vi "Check Moved File.vi"(7 "Baseline Directory":path, 8 "error in":errorcluster, 10 "Target":string, 11 "File Info in":T1) -> (0 "error out":errorcluster, 3 "File Info out":T1)   [LabVIEW 2020, in "Peer Review.lvclass"]
uses:
  Peer Review.lvclass
  TypeDefs/File Info.ctl
  TypeDefs/File State.ctl
  TypeDefs/VI Type.ctl
  <vilib>/security/Message Digest/API/Instances/File/SHA-256 File Checksum.vi
  <vilib>/security/Message Digest/API/NI_Message Digest API.lvlib
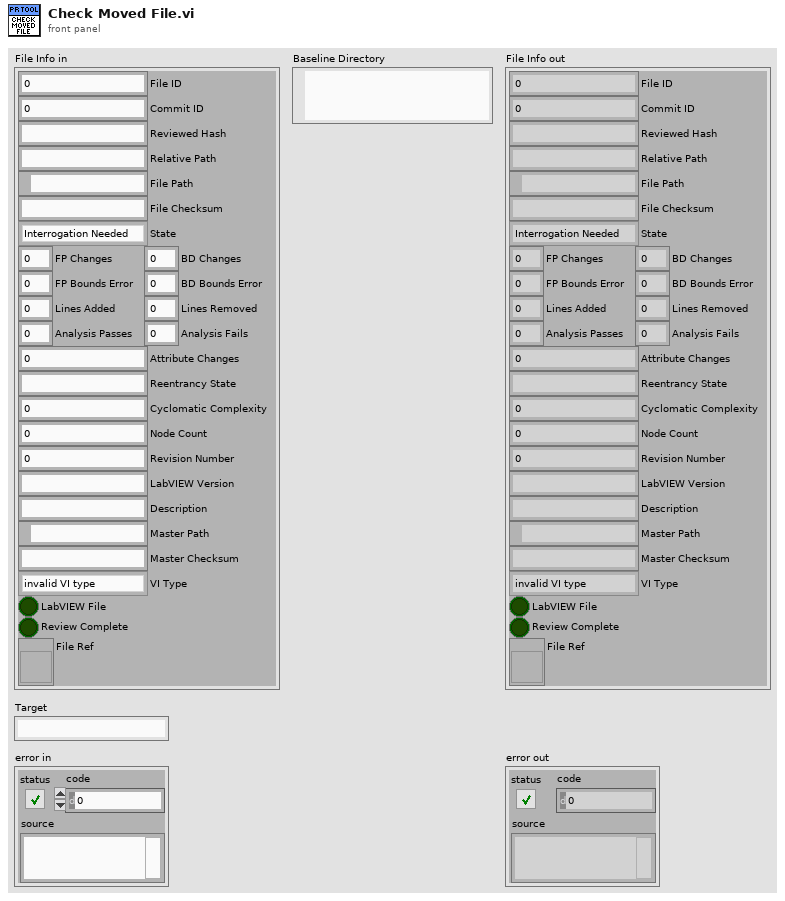
[diagram p1: front panel]
types:
  T1 = typedef "Peer Review.lvclass/File Info.ctl" = cluster{"File ID":i32, "Commit ID":i32, "Reviewed Hash":string, "Relative Path":string, "File Path":path, "File Checksum":string, "State":T2, "FP Changes":i32, "BD Changes":i32, "FP Bounds Error":dbl, "BD Bounds Error":dbl, "Lines Added":i32, "Lines Removed":i32, "Analysis Passes":i32, "Analysis Fails":i32, "Attribute Changes":i32, "Reentrancy State":string, "Cyclomatic Complexity":i32, "Node Count":i32, "Revision Number":u32, "LabVIEW Version":string, "Description":string, "Master Path":path, "Master Checksum":string, "VI Type":T3, "LabVIEW File":bool, "Review Complete":bool, "File Ref":refnum<vi>}
  T2 = typedef "Peer Review.lvclass/File State.ctl" = enum16{"Interrogation Needed", "Modified", "Deleted", "Added", "Matches Previous", "No Changes", "Moved"}
  T3 = typedef "Peer Review.lvclass/VI Type.ctl" = enum32{"invalid VI type", "Standard VI", "Control VI", "Global VI", "Polymorphic VI", "Configuration VI", "SubSystem", "Facade VI", "Method VI", "Statechart Diagram VI"}
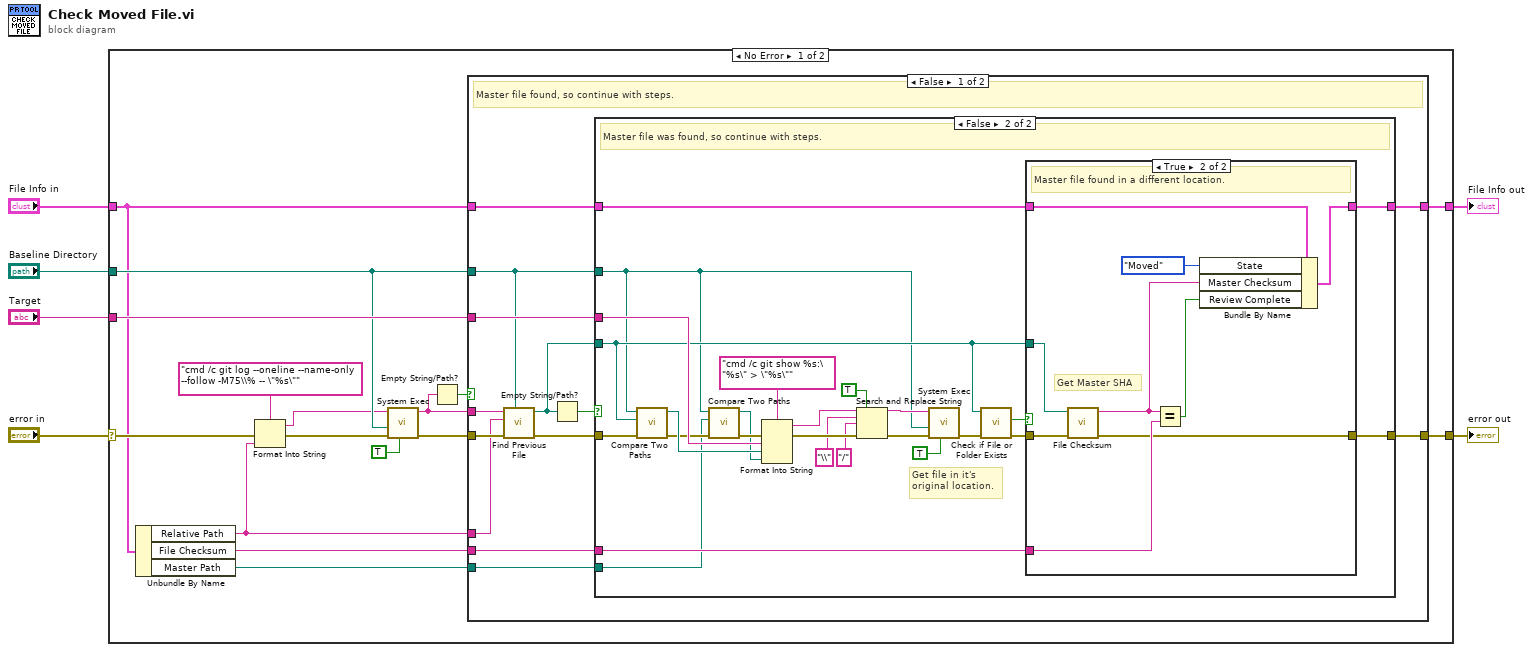
[diagram p0: block diagram]
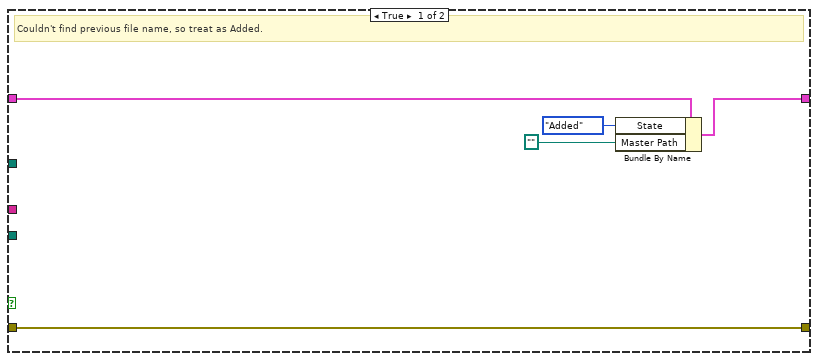
[diagram p2: hidden frame]
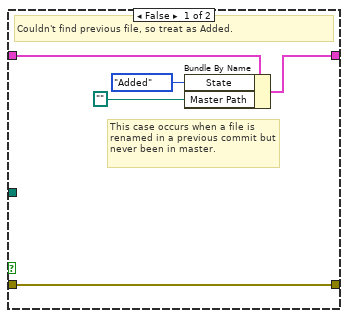
[diagram p3: hidden frame]
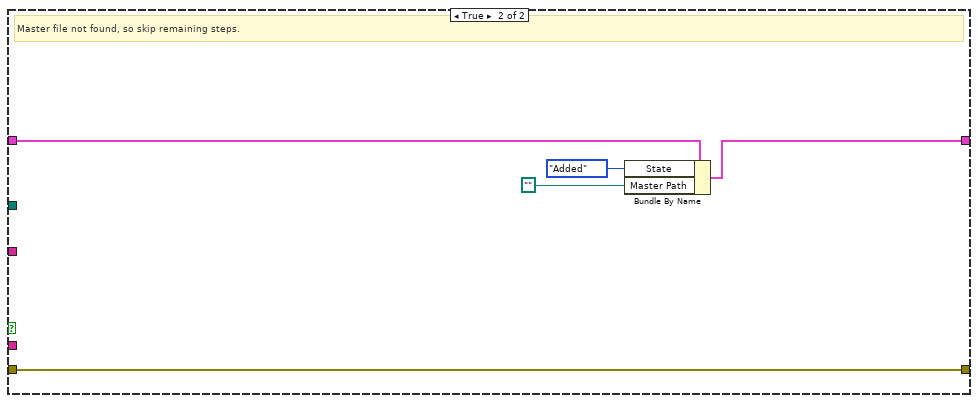
[diagram p4: hidden frame]
diagram:
  n1 = case shown="No Error" "error in" {
    selector: "error in" -> [w22 w86]
    tunnel: "Target" -> [w21 _]
    tunnel: "Baseline Directory" -> [w20 _]
    tunnel: [w13 w86] -> w3
    tunnel: "File Info in" -> [w10 w85]
    tunnel: [w9 w85] -> w1
    frame No Error {
      n2 = Unbundle By Name(w10) -> ("Relative Path"=w8:string, "File Checksum"=w11:string, "Master Path"=w7:path)
      n3 = Format Into String(format string="cmd /c git log --oneline --name-only --follow -M75\\% -- \"%s\"" ("command line"), error in=w22, w8) -> (resulting string=w15:string, error out=w18:errorcluster)  [unwired: 1 in]
      n4 = call <vilib>:"System Exec.vi"("run minimized? (F)"=TRUE, "error in (no error)"=w18, "working directory"=w20, "command line"=w15) -> ("error out"=w16:errorcluster, "standard output"=w14:string)  [unwired: 4 in, 2 out]
      n5 = Empty String/Path?(string/path=w14) -> (empty?=w12:bool)
      n6 = case shown="False" w12 {
        tunnel: w21 -> [w35 _]
        tunnel: w20 -> [w23 _]
        tunnel: w16 -> [w28 w81]
        tunnel: w14 -> [w29 _]
        tunnel: [w32 w81] -> w13
        tunnel: w11 -> [w34 _]
        tunnel: w10 -> [w30 w84]
        tunnel: [w31 w82] -> w9
        tunnel: w7 -> [w33 _]
        tunnel: w8 -> [w26 _]
        frame False {
          # "Master file found, so continue with steps."
          n7 = call "Find Previous File.vi"("Baseline Directory"=w23, "error in"=w28, "Relative Path"=w26, "Response String"=w29) -> ("error out"=w27:errorcluster, "Previous Name"=w25:path)  [unwired: 6 in]
          n8 = Empty String/Path?(string/path=w25) -> (empty?=w24:bool)
          n9 = case shown="False" w24 {
            tunnel: w35 -> [_ w49]
            tunnel: w34 -> [_ w64]
            tunnel: w33 -> [_ w42]
            tunnel: [w37 w63] -> w32
            tunnel: [w38 w62] -> w31
            tunnel: w30 -> [w39 w61]
            tunnel: w23 -> [_ w43]
            tunnel: w27 -> [w37 w48]
            tunnel: w25 -> [_ w47]
            frame True {
              # "Couldn't find previous file name, so treat as Added."
              n10 = Bundle By Name(cluster=w39, "State"=File_State."Added" ("File State"), "Master Path"=path "") -> (w38:T1)
            }
            frame False {
              # "Get file in it's\noriginal location."
              # "Master file was found, so continue with steps."
              n11 = call <vilib>:"Compare Two Paths.vi"("error in (no error)"=w48, "Path 2"=w47, "Path 1"=w43) -> ("error out"=w45:errorcluster, "Relative Path from 1 to 2"=w46:path)  [unwired: 5 in, 2 out]
              n12 = call <vilib>:"Compare Two Paths.vi"("error in (no error)"=w45, "Path 2"=w42, "Path 1"=w43) -> ("error out"=w44:errorcluster, "Relative Path from 1 to 2"=w41:path)  [unwired: 5 in, 2 out]
              n13 = Format Into String(format string="cmd /c git show %s:\"%s\" > \"%s\"", error in=w44, w49, w46, w41) -> (resulting string=w56:string, error out=w57:errorcluster)  [unwired: 1 in]
              n14 = Search and Replace String(replace all?=TRUE ("replace all? (F)"), input string=w56, search string="\\", replace string="/", error in=w57) -> (result string=w50:string, error out=w51:errorcluster)  [unwired: 3 in, 2 out]
              n15 = call <vilib>:"System Exec.vi"("run minimized? (F)"=TRUE, "error in (no error)"=w51, "working directory"=w43, "command line"=w50) -> ("error out"=w60:errorcluster)  [unwired: 4 in, 3 out]
              n16 = call <vilib>:"Check if File or Folder Exists.vi"("error in (no error)"=w60, "path"=w47) -> ("error out"=w59:errorcluster, "file or folder exists?"=w58:bool)  [unwired: 7 in, 1 out]
              n17 = case shown="True" w58 {
                tunnel: w64 -> [_ w79]
                tunnel: [w68 w72] -> w63
                tunnel: [w69 w78] -> w62
                tunnel: w61 -> [w67 w75]
                tunnel: w59 -> [w68 w77]
                tunnel: w47 -> [_ w76]
                frame False {
                  # "This case occurs when a file is renamed in a previous commit but never been in master."
                  # "Couldn't find previous file, so treat as Added."
                  n18 = Bundle By Name(cluster=w67, "State"=File_State."Added" ("File State"), "Master Path"=path "") -> (w69:T1)
                }
                frame True {
                  # "Get Master SHA"
                  # "Master file found in a different location."
                  n19 = call-poly <vilib>:"File Checksum.vi"("error in"=w77, "path"=w76) -> ("error out"=w72:errorcluster, "digest"=w74:string)  [unwired: 8 in]
                  n20 = Equal?(x=w74, y=w79) -> (x = y?=w73:bool)
                  n21 = Bundle By Name(cluster=w75, "State"=File_State."Moved" ("File State"), "Master Checksum"=w74, "Review Complete"=w73) -> (w78:T1)
                }
              }
            }
          }
        }
        frame True {
          # "Master file not found, so skip remaining steps."
          n22 = Bundle By Name(cluster=w84, "State"=File_State."Added" ("File State"), "Master Path"=path "") -> (w82:T1)
        }
      }
    }
    frame Error {
    }
  }
  "error out" <- w3
  "File Info out" <- w1
